vi "BasicRead.vi"() -> ()   [LabVIEW 2020]
panel:
  out "text":string
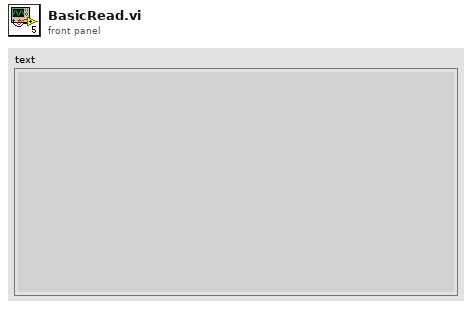
[diagram p1: front panel]
types:
  T1 = enum16{"open", "replace", "create", "open or create", "replace or create", "replace or create with confirmation"}
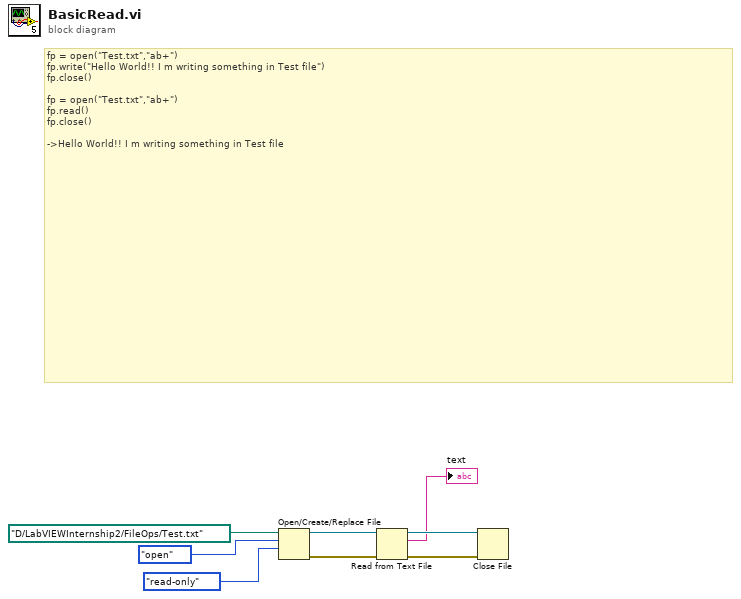
[diagram p0: block diagram]
diagram:
  # "fp = open(\"Test.txt\",\"ab+\")\nfp.write(\"Hello World!! I m writing something in Test file\")\nfp.close()\n\nfp = open(\"Test.txt\",\"ab+\")\nfp.read()\nfp.close()\n\n->Hello World!! I m writing something in Test file"
  n1 = Open/Create/Replace File(file path (use dialog)=path "D:/LabVIEWInternship2/FileOps/Test.txt", operation (0:open)=T1."open", access (0:read/write)=enum16{"read/write", "read-only", "write-only"}."read-only") -> (refnum out=w8:refnum<file>, error out=w7:errorcluster)  [unwired: 3 in, 1 out]
  n2 = Read from Text File(file (use dialog)=w8, error in=w7) -> (refnum out=w6:refnum<file>, text=→"text":string, error out=w5:errorcluster)  [unwired: 2 in, 1 out]
  n3 = Close File(refnum=w6, error in=w5) -> ()  [unwired: 2 out]
